vi "Wrap Angle (array).vi"(7 "angle units":T1 items=["radian in, radian out", "radian in, degree out", "degree in, degree out", "degree in, radian out"], 10 "angle range":T2=1 items=["none", "-180 to 180 (-pi to pi)", "0 to 360 (0 to 2pi)"], 11 "Angle In":dbl[](array[numeric])) -> (0 "error":i32, 3 "Angle Out":dbl[](array[numeric]))   [LabVIEW 2020, in "NI_AAL_Angle.lvlib"]
doc: "Wraps the input angle to a value within the range you specify with <B>angle range</B>.\n\nWire data to any of the angle inputs to determine the polymorphic instance to use or manually select the instance."
uses:
  <vilib>/Analysis/NI_AAL_Angle.lvlib
  <vilib>/Analysis/coordinate.llb/Angle Range (Degree).ctl
  <vilib>/Analysis/coordinate.llb/Angle Units.ctl
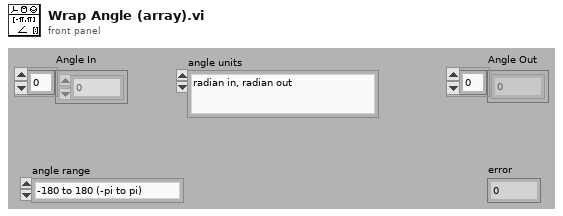
[diagram p1: front panel]
types:
  T1 = typedef "NI_AAL_Angle.lvlib/Angle Units.ctl" = i32
  T2 = typedef "NI_AAL_Angle.lvlib/Angle Range (Degree).ctl" = u16
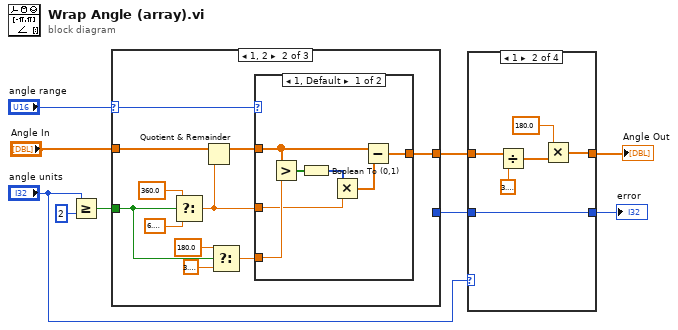
[diagram p0: block diagram]
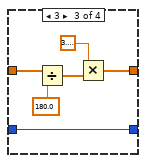
[diagram p3: hidden frame]
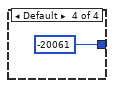
[diagram p4: hidden frame]
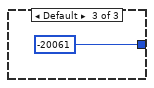
[diagram p7: hidden frame]
diagram:
  n1 = Greater Or Equal?(x="angle units", y=2) -> (x >= y?=w7:bool)
  n2 = case shown="1, 2" "angle range" {
    selector: "angle range" -> [_ w18 _]
    tunnel: "Angle In" -> [w10 w20 _]
    tunnel: [w10 w19 _] -> w6
    tunnel: [_ _ -20061] -> w5
    tunnel: w7 -> [_ w14 _]
    frame 0 {
    }
    frame 1, 2 {
      n3 = Select(t=360.0, s=w14, f=6.283185307179586) -> (s? t:f=w15:dbl)
      n4 = Quotient & Remainder(x=w20, y=w15) -> (x-y*floor(x/y)=w21:dbl[])  [unwired: 1 out]
      n5 = Select(t=180.0, s=w14, f=3.141592653589793) -> (s? t:f=w11:dbl)
      n6 = case shown="1, Default" w18 {
        tunnel: w21 -> [w28 w29]
        tunnel: [w27 w29] -> w19
        tunnel: w15 -> [w23 _]
        tunnel: w11 -> [w26 _]
        frame 1, Default {
          n7 = Greater?(x=w28, y=w26) -> (0:w25:bool[])
          n8 = Boolean To (0,1)(Boolean=w25) -> (0, 1=w24:i16[])
          n9 = Multiply(x=w24, y=w23) -> (x*y=w22:dbl[])
          n10 = Subtract(x=w28, y=w22) -> (x-y=w27:dbl[])
        }
        frame 2 {
        }
      }
    }
    frame Default {
    }
  }
  n11 = case shown="1" "angle units" {
    tunnel: w6 -> [w31 w37 w42 _]
    tunnel: w5 -> [w32 w38 w44 _]
    tunnel: [w32 w38 w44 -20061] -> w3
    tunnel: [w31 w35 w41 _] -> w1
    frame 0, 2 {
    }
    frame 1 {
      n12 = Divide(x=w37, y=3.141592653589793) -> (x/y=w34:dbl[])
      n13 = Multiply(x=180.0, y=w34) -> (x*y=w35:dbl[])
    }
    frame 3 {
      n14 = Divide(x=w42, y=180.0 ("x")) -> (x/y=w43:dbl[])
      n15 = Multiply(x=3.141592653589793, y=w43) -> (x*y=w41:dbl[])
    }
    frame Default {
    }
  }
  "error" <- w3
  "Angle Out" <- w1
